vi "draw.vi"(0 "reference":refnum<class "ActorNode.lvclass">, 1 "graphics":refnum<class "Graphics.lvclass">, 5 "error in (no error)":errorcluster) -> (14 "reference out":refnum<class "ActorNode.lvclass">, 19 "error out":errorcluster)   [LabVIEW 2014, in "ActorNode.lvclass"]
doc: "public void draw(Graphics2D g2, Point2D p, Point2D q)"
uses:
  <resource>/Framework/Providers/Open_GDS/UML/ActorNode_class/ActorNode.lvclass
  <resource>/Framework/Providers/Open_GDS/UML/Graphics_class/Graphics.lvclass
  <resource>/Framework/Providers/Open_GDS/UML/General/Point/Point Point2D.ctl
  <resource>/Framework/Providers/Open_GDS/UML/MultiLineString_class/MultiLineString.lvclass
  <resource>/Framework/Providers/Open_GDS/UML/RectangularNode_class/RectangularNode.lvclass
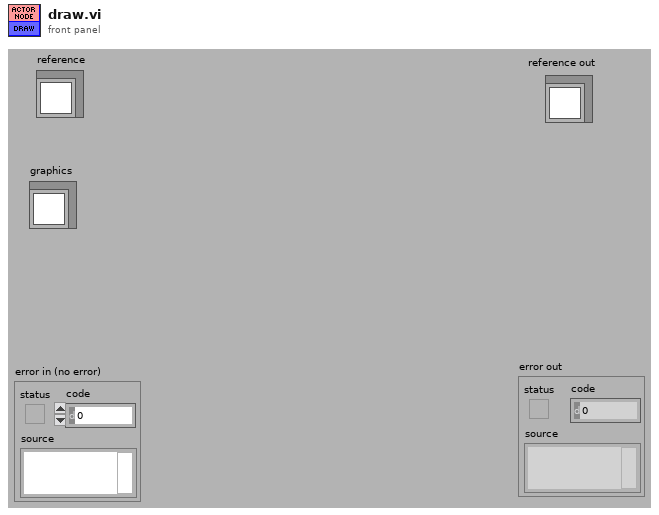
[diagram p1: front panel]
types:
  T1 = typedef "Point Point2D.ctl" = cluster{"x":dbl, "y":dbl}
  T2 = typedef "ActorNode.lvclass/ObjectAttributes.ctl" = cluster{"name":refnum<class "MultiLineString.lvclass">, "DEFAULT_WIDTH":i32, "DEFAULT_HEIGHT":i32, "DEFAULT_GAP":i32}
  T3 = typedef "RectangularNode.lvclass/ObjectAttributes.ctl" = cluster{"bounds":T4}
  T4 = typedef "Rectangle Rectangle2D.ctl" = cluster{"x":dbl, "y":dbl, "width":dbl, "height":dbl}
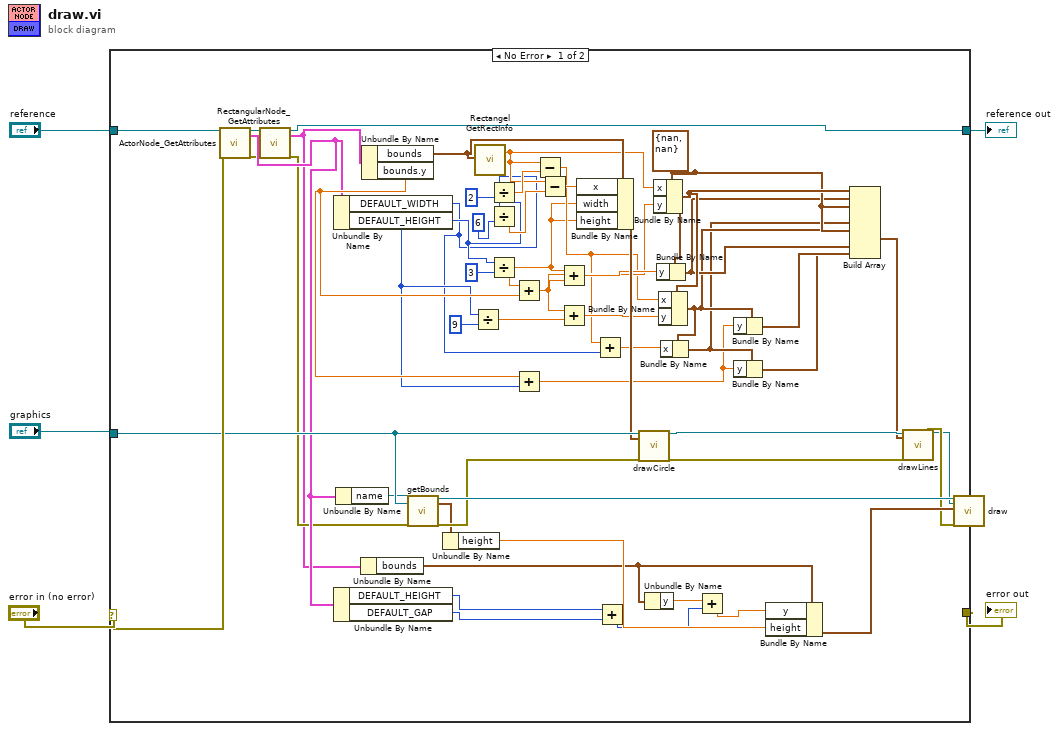
[diagram p0: block diagram]
diagram:
  n1 = case shown="No Error" "error in (no error)" {
    selector: "error in (no error)" -> [w58 w61]
    tunnel: "reference" -> [w60 w62]
    tunnel: [w59 w61] -> w4
    tunnel: [w7 w62] -> w3
    tunnel: "graphics" -> [w57 _]
    frame No Error {
      w34 = T1 {"x"=nan, "y"=nan} ("point2D")
      n2 = call <resource>:"ActorNode_GetAttributes.vi"("reference in"=w60, "error in (no error)"=w58) -> ("reference out"=w10:refnum<class "ActorNode.lvclass">, "Data"=w11:T2, "error out"=w9:errorcluster)  [unwired: 1 in, 14 out]
      n3 = call <resource>:"RectangularNode_GetAttributes.vi"("reference in"=w10, "error in (no error)"=w9) -> ("reference out"=w7:refnum<class "ActorNode.lvclass">, "Data"=w6:T3, "error out"=w8:errorcluster)  [unwired: 14 in, 1 out]
      n4 = Unbundle By Name(w11) -> ("DEFAULT_WIDTH"=w12:i32, "DEFAULT_HEIGHT"=w20:i32)
      n5 = Unbundle By Name(w11) -> ("DEFAULT_HEIGHT"=w51:i32, "DEFAULT_GAP"=w52:i32)
      n6 = Unbundle By Name(w11) -> ("name"=w56:refnum<class "MultiLineString.lvclass">)
      n7 = Unbundle By Name(w6) -> ("bounds"=w26:T4)
      n8 = Unbundle By Name(w6) -> ("bounds"=w48:T4, "bounds.y"=w21:dbl)
      n9 = call-dynamic "getBounds.vi"("reference"=w56, "graphics"=w57, "error in (no error)"=w8) -> ("reference out"=w55:refnum<class "MultiLineString.lvclass">, "bounds"=w53:T4, "error out"=w54:errorcluster)  [unwired: 14 in]
      n10 = Unbundle By Name(w53) -> ("height"=w50:dbl)
      n11 = Divide(x=w20, y=9) -> (x/y=w40:dbl)
      n12 = call <resource>:"Rectangel GetRectInfo.vi"("bounds"=w48) -> ("centerX"=w15:dbl)  [unwired: 1 in, 17 out]
      n13 = Divide(x=w12, y=2) -> (x/y=w17:dbl)
      n14 = Divide(x=w20, y=6) -> (x/y=w46:dbl)
      n15 = Divide(x=w20, y=3) -> (x/y=w13:dbl)
      n16 = Add(x=w13, y=w21) -> (x+y=w31:dbl)
      n17 = Add(x=w21, y=w20) -> (x+y=w19:dbl)
      n18 = Subtract(x=w15, y=w17) -> (x-y=w14:dbl)
      n19 = Subtract(x=w15, y=w46) -> (x-y=w16:dbl)
      n20 = Add(x=w13, y=w31) -> (x+y=w39:dbl)
      n21 = Add(x=w31, y=w40) -> (x+y=w35:dbl)
      n22 = Bundle By Name(cluster=w48, "x"=w16, "width"=w13, "height"=w13) -> (w44:T4)
      n23 = Add(x=w14, y=w12) -> (x+y=w22:dbl)
      n24 = Add(x=w51, y=w52) -> (x+y=w24:i32)
      n25 = call-dynamic "drawCircle.vi"("reference"=w57, "rectangle"=w44, "error in (no error)"=w54) -> ("reference out"=w43:refnum<class "Graphics.lvclass">, "error out"=w42:errorcluster)  [unwired: 15 in]
      n26 = Unbundle By Name(w26) -> ("y"=w25:dbl)
      n27 = Bundle By Name(cluster=w34, "x"=w15, "y"=w31) -> (w38:T1)
      n28 = Bundle By Name(cluster=w38, "y"=w39) -> (w33:T1)
      n29 = Bundle By Name(cluster=w38, "x"=w14, "y"=w35) -> (w32:T1)
      n30 = Bundle By Name(cluster=w32, "x"=w22) -> (w30:T1)
      n31 = Add(x=w25, y=w24) -> (x+y=w23:dbl)
      n32 = Bundle By Name(cluster=w32, "y"=w19) -> (w29:T1)
      n33 = Bundle By Name(cluster=w30, "y"=w19) -> (w28:T1)
      n34 = Bundle By Name(cluster=w26, "y"=w23, "height"=w50) -> (w49:T4)
      n35 = Build Array(w38, w33, w34, w32, w30, w34, w29, w33, w28) -> (w27:T1[])
      n36 = call <resource>:"drawLines.vi"("reference"=w43, "points"=w27, "error in (no error)"=w42) -> ("reference out"=w36:refnum<class "Graphics.lvclass">, "error out"=w37:errorcluster)  [unwired: 4 in, 11 out]
      n37 = call-dynamic "draw.vi"("reference"=w55, "graphics"=w36, "bounds"=w49, "error in (no error)"=w37) -> ("error out"=w59:errorcluster)  [unwired: 14 in, 1 out]
    }
    frame Error {
    }
  }
  "reference out" <- w3
  "error out" <- w4
